vi "Oscilloscope.vi"() -> ()   [LabVIEW 2017]
uses:
  <vilib>/express/express analysis/Spectral/Block/exnSpectralBlock spectral measurements RMS poly.vi
  <vilib>/express/express analysis/Spectral/Block/exnSpectralBlock spectral measurements RMS DDT.vi
  <vilib>/express/express analysis/Spectral/XNode/ExpressSpectralMeasurementsBlockNode.xnode
panel:
  out "Time":dynamicdata(graph) caption="Data"
  out "Frequency":dbl
  out "Spectrum":dynamicdata(graph)
  in  "stop":bool
  # "Developed by Vincent Claes"
  # "Hz"
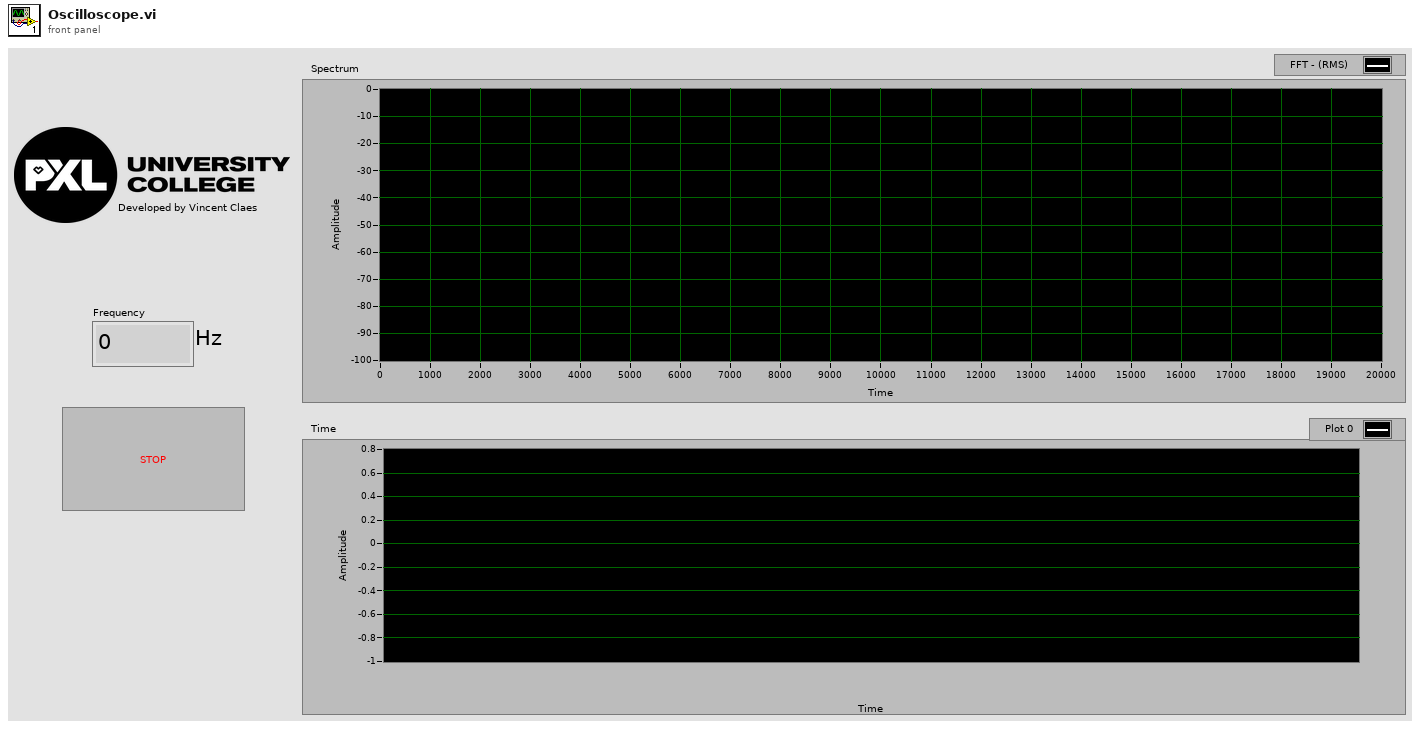
[diagram p1: front panel]
types:
  T1 = cluster{"averaging mode":u16, "weighting mode":u16, "number of averages":u32}
  T2 = cluster{"dB On (F)":bool, "unwrap phase (F)":bool, "convert to degree (F)":bool}
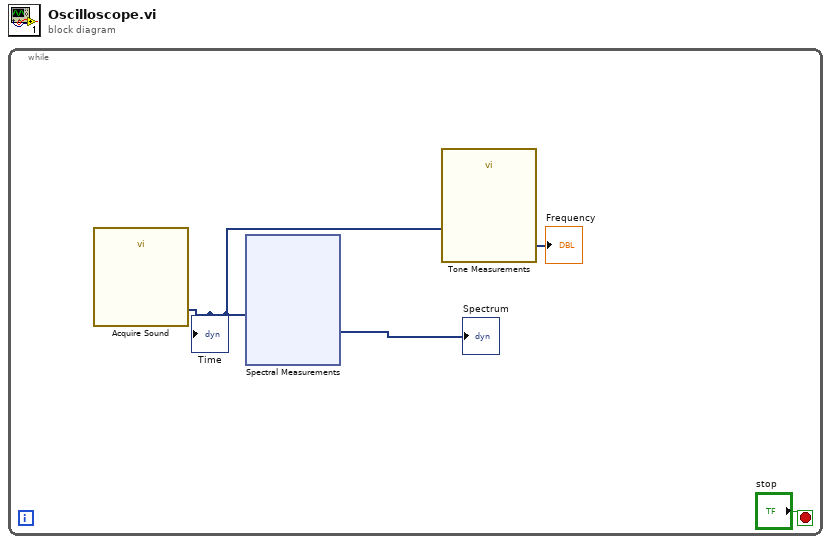
[diagram p0: block diagram]
diagram:
  n1 = while {
    stop <- "stop" stop-if-true
    n2 = call "Acquire Sound"() -> ("Data"=w2:dynamicdata)  [unwired: 18 in, 1 out]
    "Time" <- w2
    n3 = xnode "Spectral Measurements"("Signals"=w2) -> ("FFT - (RMS)"=→"Spectrum":dynamicdata)  [unwired: 1 in, 2 out]
    n4 = call "Tone Measurements"("Signals"=w2) -> ("Frequency"=→"Frequency":dynamicdata)  [unwired: 9 in, 1 out]
  }
